vi "Get Output Array.vi"(8 "error in":errorcluster, 11 "Device Ref in":T1 format="%.0x") -> (0 "error out":errorcluster, 1 "Energy Index":i32, 2 "Voltage Index":i32, 3 "Array":string[](array[string]))   [LabVIEW 2021, in "G5 Regatron Custom Device Engine.lvlib"]
uses:
  G5 Regatron Custom Device Engine.lvlib
  <vilib>/NI VeriStand/Custom Device API/Custom Device Item Ref.ctl
  <userlib>/_OpenG.lib/array/array.llb/Search 1D Array (String)__ogtk.vi
  <vilib>/NI VeriStand/Custom Device API/Custom Device API.lvlib
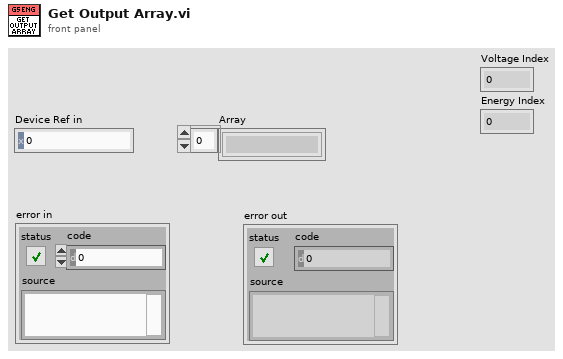
[diagram p1: front panel]
types:
  T1 = typedef "Custom Device API.lvlib/Custom Device Item Ref.ctl" = u64
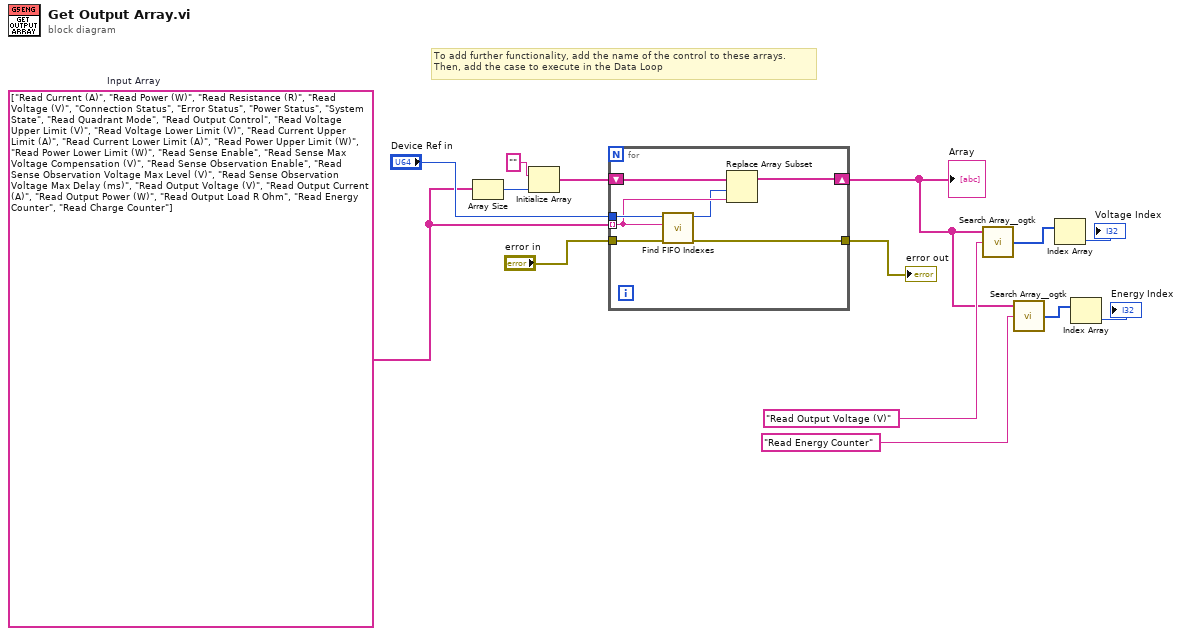
[diagram p0: block diagram]
diagram:
  w13 = string[] ["Read Current (A)", "Read Power (W)", "Read Resistance (R)", "Read Voltage (V)", "Connection Status", "Error Status", "Power Status", "System State", "Read Quadrant Mode", "Read Output Control", "Read Voltage Upper Limit (V)", "Read Voltage Lower Limit (V)", "Read Current Upper Limit (A)", "Read Current Lower Limit (A)", "Read Power Upper Limit (W)", "Read Power Lower Limit (W)", "Read Sense Enable", "Read Sense Max Voltage Compensation (V)", "Read Sense Observation Enable", "Read Sense Observation Voltage Max Level (V)", "Read Sense Observation Voltage Max Delay (ms)", "Read Output Voltage (V)", "Read Output Current (A)", "Read Output Power (W)", "Read Output Load R Ohm", "Read Energy Counter", "Read Charge Counter"]  # Input Array
  # "To add further functionality, add the name of the control to these arrays.\nThen, add the case to execute in the Data Loop"
  n1 = Array Size(array=w13) -> (size(s)=w9:i32)
  n2 = Initialize Array("", w9) -> (w11:string[])
  n3 = for {
    tunnel: "Device Ref in" -> [w21]
    tunnel: w13 -> [w16] mode=indexing
    tunnel: "error in" -> [w20]
    tunnel: [w19] -> w12
    shift-right: [w17] -> w5
    shift-left: w11 -> [w18]
    n4 = call "Find FIFO Indexes.vi"("error in"=w20, "Item Name"=w16, "Custom Device Ref in"=w21) -> ("error out"=w19:errorcluster, "Index"=w15:i32)  [unwired: 7 in]
    n5 = Replace Array Subset(array=w18, new element=w16, index=w15) -> (w17:string[])
  }
  "error out" <- w12
  "Array" <- w5
  n6 = call-poly <userlib>:"Search Array__ogtk.vi"("Array"=w5, "Element Data"="Read Output Voltage (V)" ("String")) -> ("Indices of Elements"=w4:i32[])  [unwired: 7 in]
  n7 = call-poly <userlib>:"Search Array__ogtk.vi"("Array"=w5, "Element Data"="Read Energy Counter" ("String")) -> ("Indices of Elements"=w2:i32[])  [unwired: 7 in]
  n8 = Index Array(array=w4) -> (element=→"Voltage Index":i32)  [unwired: 1 in]
  n9 = Index Array(array=w2) -> (element=→"Energy Index":i32)  [unwired: 1 in]
